vi "start subscription.vi"(8 "error in":errorcluster, 10 "subject":string, 11 "NATS Client":refnum<class "NATS Client.lvclass">) -> (0 "error out":errorcluster, 3 "NATS Subscription":refnum<class "NATS Subscription.lvclass">)   [LabVIEW 2024, in "NAT Subscription.lvlib" / "NATS Subscription.lvclass"]
uses:
  NATS Subscription.lvclass
  NATS Client/NATS Client.lvclass
  Controls/nats message.ctl
  Controls/msg type.ctl
  NATS Subscription.lvclass/NATS Subscription.ctl
  set subject.vi
  set id.vi
  set reply queue.vi
  NATS Core.lvlib
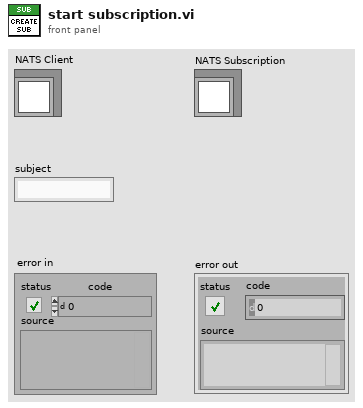
[diagram p1: front panel]
types:
  T1 = typedef "NATS Core.lvlib/nats message.ctl" = cluster{"subject":string, "payload":string, "sub id":string, "reply-to":string, "headers":string, "type":T2, "received":timestamp}
  T2 = typedef "NATS Core.lvlib/msg type.ctl" = enum16{"Undefined", "MSG", "HMSG", "+OK", "PING", "PONG", "-ERR", "INFO"}
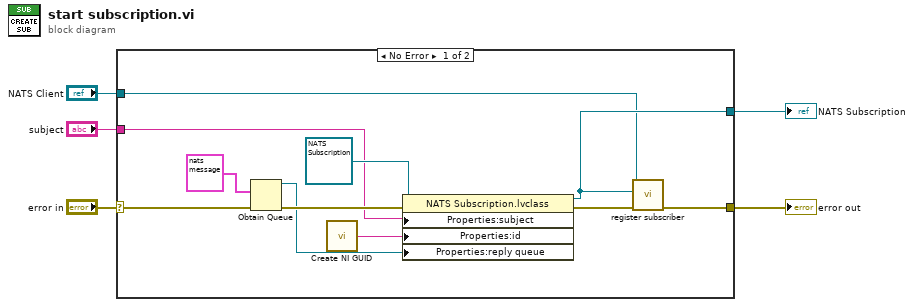
[diagram p0: block diagram]
diagram:
  n1 = case shown="No Error" "error in" {
    selector: "error in" -> [w16 w17]
    tunnel: "subject" -> [w11 _]
    tunnel: [w14 w17] -> w4
    tunnel: [w7 _] -> w2
    tunnel: "NATS Client" -> [w6 _]
    frame No Error {
      n2 = Obtain Queue(element data type=T1 {"subject"="", "payload"="", "sub id"="", "reply-to"="", "headers"="", "type"=enum."Undefined", "received"=timestamp(0 s since 1904-01-01)} ("nats message"), error in (no error)=w16) -> (queue out=w8:refnum<queue>, error out=w15:errorcluster)  [unwired: 3 in, 1 out]
      n3 = call <vilib>:"Create NI GUID.vi"() -> ("NI GUID"=w10:string)
      n4 = property class="NATS Subscription.lvclass"(reference=refnum<class "NATS Subscription.lvclass"> refnum ("NATS Core.lvlib:NATS Subscription.lvclass"), error in=w15, "Properties:subject"=w11, "Properties:id"=w10, "Properties:reply queue"=w8) -> (reference out=w7:refnum<class "NATS Subscription.lvclass">, error out=w13:errorcluster)
      n5 = call "register subscriber.vi"("error in"=w13, "NATS Subscription"=w7, "NATS Client in"=w6) -> ("error out"=w14:errorcluster)  [unwired: 7 in, 1 out]
    }
    frame Error {
    }
  }
  "error out" <- w4
  "NATS Subscription" <- w2
